vi "Update Property.vi"(8 "error in (no error)":errorcluster, 9 "Value":variant, 10 "Name":string, 11 "IntegerPanel in":refnum<class "IntegerPanel.lvclass">) -> (0 "error out":errorcluster, 3 "IntegerPanel out":refnum<class "IntegerPanel.lvclass">)   [LabVIEW 2020, in "Conditum-Tools.lvlib" / "IntegerPanel.lvclass"]
uses:
  IntegerPanel.lvclass
  IntegerPanel.lvclass/IntegerPanel.ctl
  Conditum-Clone/Columns/Integer/Integer.lvclass
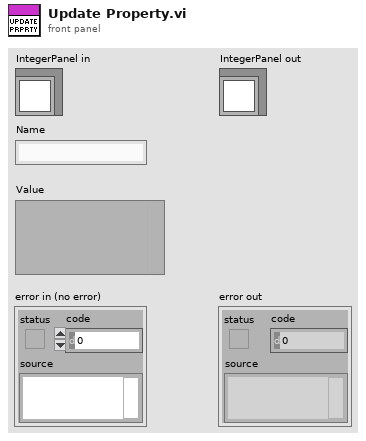
[diagram p1: front panel]
types:
  T1 = typedef "Conditu2.lvlib/Columns.lvlib/Integer.lvclass/Definition.ctl" = cluster{"Default":i64}
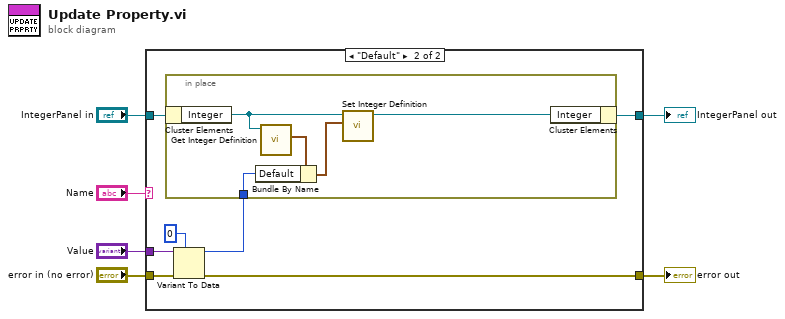
[diagram p0: block diagram]
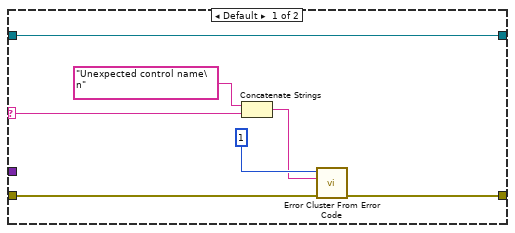
[diagram p2: hidden frame]
diagram:
  n1 = case shown="\"Default\"" "Name" {
    selector: "Name" -> [w9 _]
    tunnel: "Value" -> [_ w20]
    tunnel: "IntegerPanel in" -> [w7 w16]
    tunnel: "error in (no error)" -> [w13 w18]
    tunnel: [w12 w17] -> w1
    tunnel: [w7 w14] -> w2
    frame Default {
      n2 = Concatenate Strings("Unexpected control name\n" ("format string"), w9) -> (w8:string)
      n3 = call <vilib>:"Error Cluster From Error Code.vi"("error in (no error)"=w13, "error message (\"\")"=w8, "error code (0)"=1) -> ("error out"=w12:errorcluster)  [unwired: 6 in]
    }
    frame "Default" {
      n4 = Variant To Data(error in=w18, type=i64 0, Variant=w20) -> (data=w15:i64, error out=w17:errorcluster)
      n5 = in-place {
        in-place-border: w15 -> [w24]
        n6 = in-place-cluster #1(w16) -> ("Integer"=w23:refnum<class "Integer.lvclass">)
        n7 = call "Get Integer Definition.vi"("Integer in"=w23) -> ("Definition"=w25:T1)  [unwired: 10 in]
        n8 = Bundle By Name(cluster=w25, "Default"=w24) -> (w22:T1)
        n9 = call "Set Integer Definition.vi"("Integer Definition"=w22, "Integer in"=w23) -> ("Integer out"=w21:refnum<class "Integer.lvclass">)  [unwired: 9 in]
        n10 = in-place-cluster #1("Integer"=w21) -> (w14:refnum<class "IntegerPanel.lvclass">)
      }
    }
  }
  "error out" <- w1
  "IntegerPanel out" <- w2
